vi "Read Switching Function Configuration.vi"(7 "function":u16(ring)=1 items=["1"=1, "2"=2, "3"=3, "4"=4, "5"=5, "6"=6], 8 "error in (no error)":errorcluster, 11 "VGC in":refnum<class "PL Inficon VGC.lvclass">) -> (0 "error out":errorcluster, 1 "thresholds":cluster{"lower":dbl, "upper":dbl}, 2 "mode":u16(ring)=1 items=["off", "on", "channel 1", "channel 2", "channel 3"], 3 "VGC out":refnum<class "PL Inficon VGC.lvclass">)   [LabVIEW 2015, in "PL Inficon VGC.lvclass"]
doc: "Reads switching function configuration."
uses:
  PL Inficon VGC.lvclass
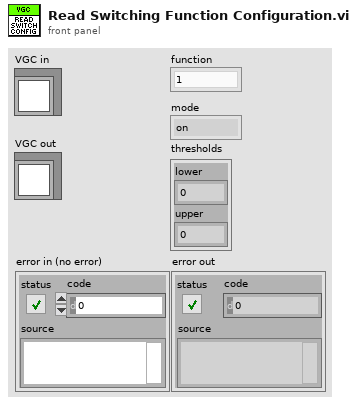
[diagram p1: front panel]
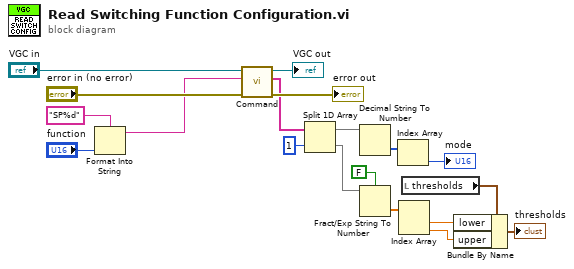
[diagram p0: block diagram]
diagram:
  n1 = Format Into String(format string="SP%d", "function") -> (resulting string=w7:string)  [unwired: 2 in, 1 out]
  n2 = call "Command.vi"("error in (no error)"="error in (no error)", "command"=w7, "VGC in"="VGC in") -> ("error out"=→"error out":errorcluster, "response data"=w14:string[], "VGC out"=→"VGC out":refnum<class "PL Inficon VGC.lvclass">)  [unwired: 6 in]
  n3 = Split 1D Array(array=w14, index=1) -> (first subarray=w12:string[], second subarray=w11:string[])
  n4 = Decimal String To Number(string=w12) -> (number=w6:i32[])  [unwired: 2 in, 1 out]
  n5 = Fract/Exp String To Number(use system decimal point (T)=FALSE, string=w11) -> (number=w10:dbl[])  [unwired: 2 in, 1 out]
  n6 = Index Array(array=w6) -> (element=→"mode":i32)  [unwired: 1 in]
  n7 = Index Array(array=w10) -> (element #1=w3:dbl, element #2=w2:dbl)  [unwired: 2 in]
  n8 = local read "thresholds"() -> (w4:cluster{"lower":dbl, "upper":dbl})
  n9 = Bundle By Name(cluster=w4, "lower"=w3, "upper"=w2) -> (→"thresholds":cluster{"lower":dbl, "upper":dbl})
